vi "Initialize Output Channel Page.vi"(8 "error in":errorcluster, 11 "Node Ptr":T1 format="%.0x") -> (0 "error out":errorcluster, 2 "Channel Settings Table":string[][](array[string]), 3 "Node Ptr out":T1=18446744073709551615 format="%.0x", 5 "BaseNodeType":refnum<k24>)   [LabVIEW 2026]
uses:
  <vilib>/NI VeriStand/Custom Device API/Custom Device Item Ref.ctl
  NationalInstruments.VeriStand.SystemStorage
  <vilib>/NI VeriStand/Custom Device API/Custom Device API.lvlib
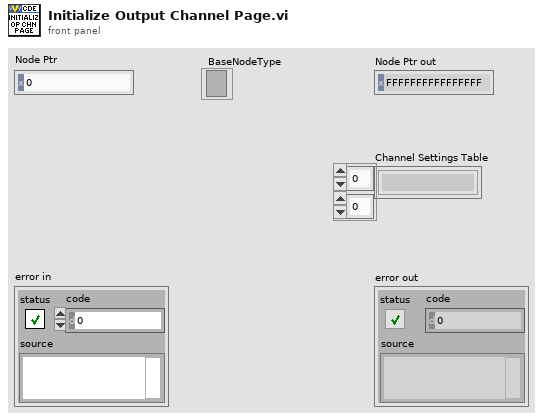
[diagram p1: front panel]
types:
  T1 = typedef "Custom Device API.lvlib/Custom Device Item Ref.ctl" = u64
  T2 = typedef "ChannelSettings.ctl" = cluster{"IsWritable":bool, "Units":string, "Default Value":dbl, "IsFaultable":bool, "IsScalable":bool}
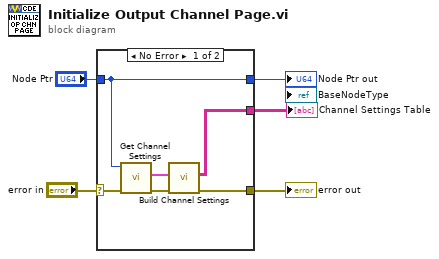
[diagram p0: block diagram]
diagram:
  n1 = case shown="No Error" "error in" {
    selector: "error in" -> [w10 w13]
    tunnel: "Node Ptr" -> [w8 w12]
    tunnel: [w6 w13] -> w3
    tunnel: [w7 _] -> w1
    tunnel: [w8 w12] -> w2
    frame No Error {
      n2 = call "Get Channel Settings.vi"("error in"=w10, "Node Ptr"=w8) -> ("error out"=w11:errorcluster, "Channel Settings"=w9:T2)  [unwired: 7 in, 1 out]
      n3 = call "Build Channel Settings.vi"("error in"=w11, "Channel Settings"=w9) -> ("error out"=w6:errorcluster, "Channel Settings Table"=w7:string[][])  [unwired: 8 in]
    }
    frame Error {
    }
  }
  "error out" <- w3
  "Node Ptr out" <- w2
  "Channel Settings Table" <- w1
